vi "Coord window-Get coordinates from top level.vi"() -> (3 "Coordinates":cluster{"X":sgl, "Y":sgl, "Z":sgl})   [LabVIEW 2013]
uses:
  Global Variables/gl_UI Ctrl Refs.vi
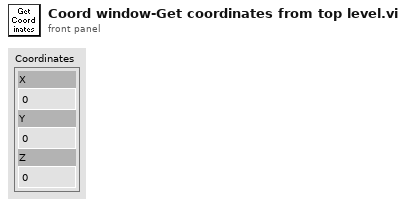
[diagram p1: front panel]
types:
  T1 = typedef "UI ctrl refs cluster.ctl" = cluster{"Top level VI path":path, "Top level VI ref":refnum<vi>, "User menu ref":refnum<k9>, "Sub Panel control":refnum<vi>, "Imaging Param Tab":refnum<vi>, "Occurrence-Start drivers":refnum<k4>, "Occurrence-Speed logging initialised":refnum<k4>, "Occurrence-XYZ stage initialised":refnum<k4>, "Exit button":refnum<vi>, "Status ind":refnum<vi>, "Return to Origin":refnum<vi>, "Speed Logging":refnum<vi>, "Time Lapse":refnum<vi>, "Live Imaging":refnum<vi>, "AOL Z Stack":refnum<vi>, "Motor Z Stack":refnum<vi>, "Funct Acq button":refnum<vi>, "Hard Shutter":refnum<vi>, "Virtual Shutter":refnum<vi>, "Laser Power":refnum<vi>, "AOL Mode":refnum<vi>, "Frame Size":refnum<vi>, "Field of View":refnum<vi>, "Dwell Time":refnum<vi>, "Zoom":refnum<vi>, "AOL Z":refnum<vi>, "Objective":refnum<vi>, "Axis":refnum<vi>, "Paths & Names":refnum<vi>, "Experiment folder path (ind.)":refnum<vi>, "Last State (Ind.)":refnum<vi>, "Laser wavelength ind (nm)":refnum<vi>, "Averages":refnum<vi>, "Angle (degrees)":refnum<vi>, "X centre":refnum<vi>, "Y centre":refnum<vi>, "Plane Mode":refnum<vi>, "# Planes":refnum<vi>, "Z Start":refnum<vi>, "Z Stop":refnum<vi>, "Z Step":refnum<vi>, "PMT 1":refnum<vi>, "PMT 2":refnum<vi>, "Stage XYZ Position":refnum<vi>, "Pockels@Z Start":refnum<vi>, "Pockels@Z Stop":refnum<vi>, "Obtain Z Start":refnum<vi>, "Obtain Z Stop":refnum<vi>, "Live stim.trig.period":refnum<vi>, "Live stim.trig.enable":refnum<vi>, "Funct. Acq. Pockels Modulation":refnum<vi>, "Enable Video Recording":refnum<vi>, "Video Record-Live Imaging":refnum<vi>, "Video Record-Funct acq":refnum<vi>, "AOL Z-stack Chirps Ready (ind)":refnum<vi>, "Center freq ind (nm)":refnum<vi>, "Logging queue (ind)":refnum<vi>, "Back aperture power (ind.)":refnum<vi>, "Power after objective (ind.)":refnum<vi>, "Switch user":refnum<vi>}
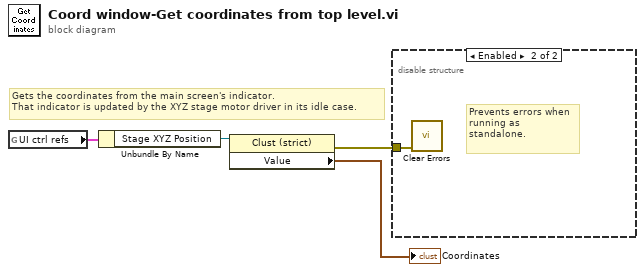
[diagram p0: block diagram]
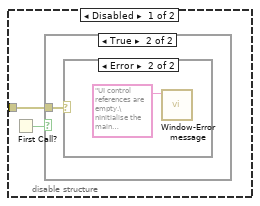
[diagram p2: hidden frame]
diagram:
  # "Gets the coordinates from the main screen's indicator.\nThat indicator is updated by the XYZ stage motor driver in its idle case."
  n1 = global read "gl_UI Ctrl Refs.vi" "UI ctrl refs"() -> (w2:T1)
  n2 = Unbundle By Name(w2) -> ("Stage XYZ Position"=w1:refnum<vi>)
  n3 = property on="Property Node" class="Clust (strict)"(reference=w1) -> (error out=w3:errorcluster, "Value"=→"Coordinates":cluster{"X":sgl, "Y":sgl, "Z":sgl})  [unwired: 1 in, 1 out]
  n4 = disable-structure shown="Enabled" {
    disable-tunnel: w3 -> [w6 w9]
    frame Disabled {
      n5 = First Call?() -> (First Call?: T/F=w5:bool)
      n6 = case shown="True" w5 {
        tunnel: w6 -> [_ w7]
        frame False {
        }
        frame True {
          n7 = case shown="Error" w7 {
            frame No Error {
            }
            frame Error {
              n8 = call "Window-Error message.vi"("Message"="UI control references are empty.\nInitialise the main application and try again." ("Error Source")) -> ()  [unwired: 10 in, 1 out]
            }
          }
        }
      }
    }
    frame Enabled {
      # "Prevents errors when running as standalone."
      n9 = call <vilib>:"Clear Errors.vi"("error in (no error)"=w9) -> ()  [unwired: 6 in, 1 out]
    }
  }
